vi "TWM Client Cmd Define QPMX.vi"(0 "handle":i32, 1 "end of packet key":string="TWM:command:EndOfPacket", 3 "timeout [ms]":i32=5000, 5 "Short circuit delay (s)":dbl=nan, 6 "Trigger polarity":enum16{"Positive", "Negative", "No change"}(ring)=enum."No change", 9 "Internal timer (s)":dbl=nan, 10 "Switch mode":T1(ring), 11 "error in":errorcluster, 12 "Sequence":bool[][](array[boolean]), 13 "Startup delay (s)":dbl=nan, 14 "Timing delays":i64[](array[numeric])) -> (4 "handle out":i32, 15 "error out":errorcluster)   [LabVIEW 2020, in "TWM Client.lvlib"]
doc: "This will define QPMX multiplexer sequence and properties. It's equivalent to manual setup of QPMX in multiplexer panel. If some inputs are not wired, particular values are not changed."
uses:
  TWM Client.lvlib
  String.vi
  EXT.vi
  2D I64.vi
  1D I64.vi
  infolib.lvlib
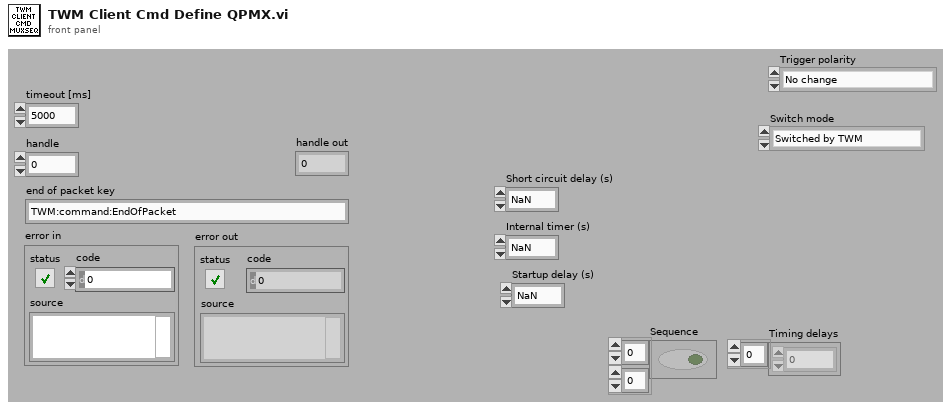
[diagram p1: front panel]
types:
  T1 = enum16{"Switched by TWM", "Switched by internal clock", "Switched by external clock", "No change"}
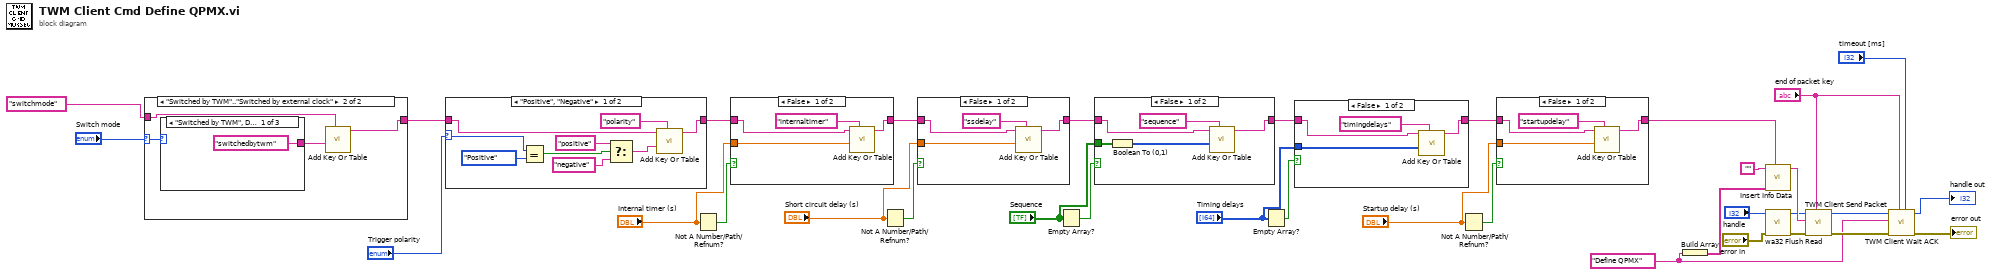
[diagram p0: block diagram]
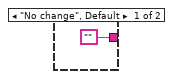
[diagram p7: hidden frame]
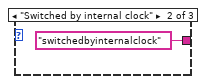
[diagram p8: hidden frame]
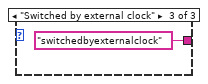
[diagram p9: hidden frame]
diagram:
  w27 = "Define QPMX" ("section name")
  n1 = case shown="\"Switched by TWM\"..\"Switched by external clock\"" "Switch mode" {
    selector: "Switch mode" -> [_ w36]
    tunnel: "switchmode" ("key description") -> [_ w38]
    tunnel: ["" w37] -> w18
    frame "No change", Default {
    }
    frame "Switched by TWM".."Switched by external clock" {
      n2 = case shown="\"Switched by TWM\", Default" w36 {
        tunnel: ["switchedbytwm" ("key description") "switchedbyinternalclock" ("key description") "switchedbyexternalclock" ("key description")] -> w39
        frame "Switched by TWM", Default {
        }
        frame "Switched by internal clock" {
        }
        frame "Switched by external clock" {
        }
      }
      n3 = call-poly "Add Key Or Table.vi"("key description"=w38, "string"=w39) -> ("info data out"=w37:string)  [unwired: 8 in, 1 out]
    }
  }
  n4 = case shown="\"Positive\", \"Negative\"" "Trigger polarity" {
    selector: "Trigger polarity" -> [w46 _]
    tunnel: w18 -> [w44 w52]
    tunnel: [w43 w52] -> w17
    frame "Positive", "Negative" {
      n5 = Equal?(x=w46, y=enum16{"Positive", "Negative", "No change"}."Positive" ("Trigger polarity")) -> (x = y?=w47:bool)
      n6 = Select(t="positive" ("key description"), s=w47, f="negative" ("key description")) -> (s? t:f=w45:string)
      n7 = call-poly "Add Key Or Table.vi"("key description"="polarity", "string"=w45, "info data"=w44) -> ("info data out"=w43:string)  [unwired: 7 in, 1 out]
    }
    frame "No change", Default {
    }
  }
  n8 = Not A Number/Path/Refnum?(number/path/refnum="Internal timer (s)") -> (NaN/Path/Refnum?=w11:bool)
  n9 = case shown="False" w11 {
    tunnel: w17 -> [w55 w57]
    tunnel: [w54 w57] -> w16
    tunnel: "Internal timer (s)" -> [w53 _]
    frame False {
      n10 = call-poly "Add Key Or Table.vi"("key description"="internaltimer", "numeric"=w53, "info data"=w55) -> ("info data out"=w54:string)  [unwired: 7 in, 1 out]
    }
    frame True {
    }
  }
  n11 = Not A Number/Path/Refnum?(number/path/refnum="Short circuit delay (s)") -> (NaN/Path/Refnum?=w9:bool)
  n12 = case shown="False" w9 {
    tunnel: w16 -> [w60 w62]
    tunnel: [w59 w62] -> w15
    tunnel: "Short circuit delay (s)" -> [w58 _]
    frame False {
      n13 = call-poly "Add Key Or Table.vi"("key description"="ssdelay", "numeric"=w58, "info data"=w60) -> ("info data out"=w59:string)  [unwired: 7 in, 1 out]
    }
    frame True {
    }
  }
  n14 = Empty Array?(array="Sequence") -> (empty?=w7:bool)
  n15 = case shown="False" w7 {
    tunnel: "Sequence" -> [w66 _]
    tunnel: w15 -> [w64 w68]
    tunnel: [w63 w68] -> w14
    frame False {
      n16 = Boolean To (0,1)(Boolean=w66) -> (0, 1=w65:i16[][])
      n17 = call-poly "Add Key Or Table.vi"("key description"="sequence", "numeric"=w65, "info data"=w64) -> ("info data out"=w63:string)  [unwired: 8 in]
    }
    frame True {
    }
  }
  n18 = Empty Array?(array="Timing delays") -> (empty?=w6:bool)
  n19 = case shown="False" w6 {
    tunnel: [w72 w73] -> w3
    tunnel: "Timing delays" -> [w70 _]
    tunnel: w14 -> [w69 w73]
    frame False {
      n20 = call-poly "Add Key Or Table.vi"("key description"="timingdelays", "numeric"=w70, "info data"=w69) -> ("info data out"=w72:string)  [unwired: 7 in, 1 out]
    }
    frame True {
    }
  }
  n21 = Not A Number/Path/Refnum?(number/path/refnum="Startup delay (s)") -> (NaN/Path/Refnum?=w2:bool)
  n22 = case shown="False" w2 {
    tunnel: w3 -> [w76 w78]
    tunnel: [w75 w78] -> w1
    tunnel: "Startup delay (s)" -> [w74 _]
    frame False {
      n23 = call-poly "Add Key Or Table.vi"("key description"="startupdelay", "numeric"=w74, "info data"=w76) -> ("info data out"=w75:string)  [unwired: 7 in, 1 out]
    }
    frame True {
    }
  }
  n24 = Build Array(w27) -> (w33:string[])
  n25 = call "Insert Info Data.vi"("info data to insert"=w1, "sections"=w33, "info data"="") -> ("info data out"=w34:string)  [unwired: 7 in, 1 out]
  n26 = call "wa32 Flush Read.vi"("error in"="error in", "handle"="handle") -> ("error out"=w23:errorcluster, "handle out"=w22:i32)  [unwired: 7 in, 1 out]
  n27 = call "TWM Client Send Packet.vi"("end of packet key"="end of packet key", "error in"=w23, "command string"=w34, "handle"=w22) -> ("error out"=w29:errorcluster, "handle out"=w26:i32)  [unwired: 6 in]
  n28 = call "TWM Client Wait ACK.vi"("timeout [ms] (3000)"="timeout [ms]", "key string"="end of packet key", "error in"=w29, "command header"=w27, "handle"=w26) -> ("error out"=→"error out":errorcluster, "handle out"=→"handle out":i32)  [unwired: 5 in]
